vi "Exp_GetTemplate.vi"(8 "error in (no error)":errorcluster, 11 "LightField Automation in":refnum<class "LightField Automation.lvclass">) -> (0 "error out":errorcluster, 2 "Setting":i32, 3 "LightField Automation out":refnum<class "LightField Automation.lvclass">)   [LabVIEW 2013, in "LightField Automation.lvclass"]
uses:
  LightField Automation.lvclass
  C:/Program Files/Princeton Instruments/LightField/PrincetonInstruments.LightFieldAddInSupportServices.dll
  Program Files/Princeton Instruments/LightField/PrincetonInstruments.LightFieldAddInSupportServices.dll
  LightField Automation.lvclass/LightField Automation.ctl
  C:/Program Files/Princeton Instruments/LightField/AddInViews/PrincetonInstruments.LightFieldViewV3.dll
  Program Files/Princeton Instruments/LightField/AddInViews/PrincetonInstruments.LightFieldViewV3.dll
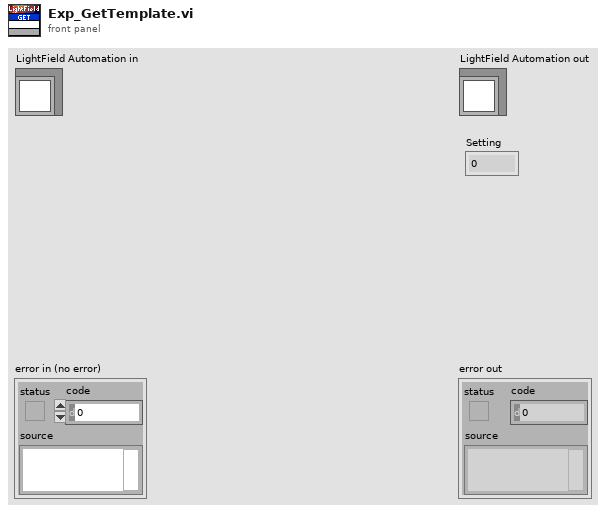
[diagram p1: front panel]
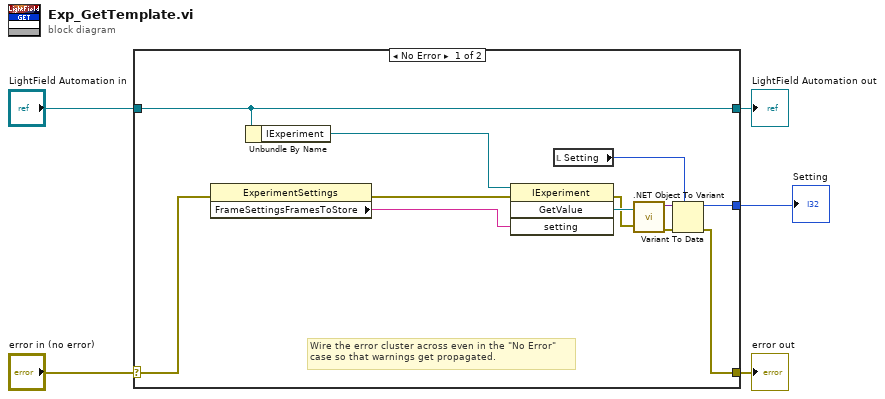
[diagram p0: block diagram]
diagram:
  n1 = case shown="No Error" "error in (no error)" {
    selector: "error in (no error)" -> [w11 w19]
    tunnel: [w7 w19] -> w4
    tunnel: [w10 w18] -> w2
    tunnel: "LightField Automation in" -> [w10 w18]
    tunnel: [w8 _] -> w1
    frame No Error {
      # "Wire the error cluster across even in the \"No Error\"\ncase so that warnings get propagated."
      n2 = property class="ExperimentSettings"(error in=w11) -> (error out=w12:errorcluster, "FrameSettingsFramesToStore"=w13:string)  [unwired: 1 in, 1 out]
      n3 = Unbundle By Name(w10) -> ("IExperiment"=w9:refnum<k24>)
      n4 = invoke class="IExperiment" method="GetValue"(reference=w9, error in=w12, "setting"=w13) -> (error out=w14:errorcluster, "GetValue"=w15:refnum<k24>)  [unwired: 1 in, 2 out]
      n5 = local read "Setting"() -> (w6:i32)
      n6 = call <vilib>:".NET Object To Variant.vi"("error in (no error)"=w14, ".NET object"=w15) -> ("error out"=w17:errorcluster, "variant"=w16:variant)
      n7 = Variant To Data(error in=w17, type=w6, Variant=w16) -> (data=w8:i32, error out=w7:errorcluster)
    }
    frame Error {
    }
  }
  "error out" <- w4
  "LightField Automation out" <- w2
  "Setting" <- w1
